vi "Prova_1.vi"(8 "error in (no error)":errorcluster, 11 "This VI":refnum<vi>) -> (0 "error out":errorcluster)   [LabVIEW 2016]
uses:
  USER32.DLL
  Program Files (x86)/VideoLAN/VLC/libvlc.dll
  System.Windows.Forms
panel:
  out "speed":dbl
  in  "PictureBox":refnum<k24>(container)
  in  "Script":string
  in  "Media Source":string="rtsp://admin:admin@192.168.1.108:554/cam/realmonitor?channel=1&subtype=1"
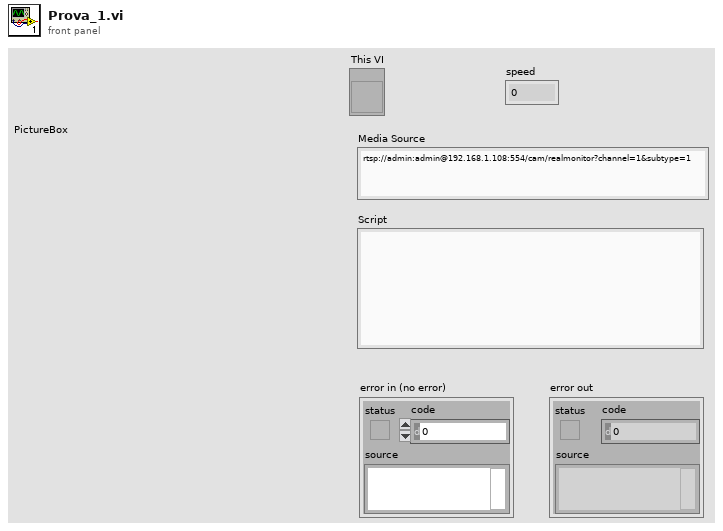
[diagram p1: front panel]
types:
  T1 = typedef "imagedata.ctl" = cluster{"image type":i32, "image depth":i32, "image":u8[], "mask":u8[], "colors":u32[], "Rectangle":cluster{"left":i16, "top":i16, "right":i16, "bottom":i16}}
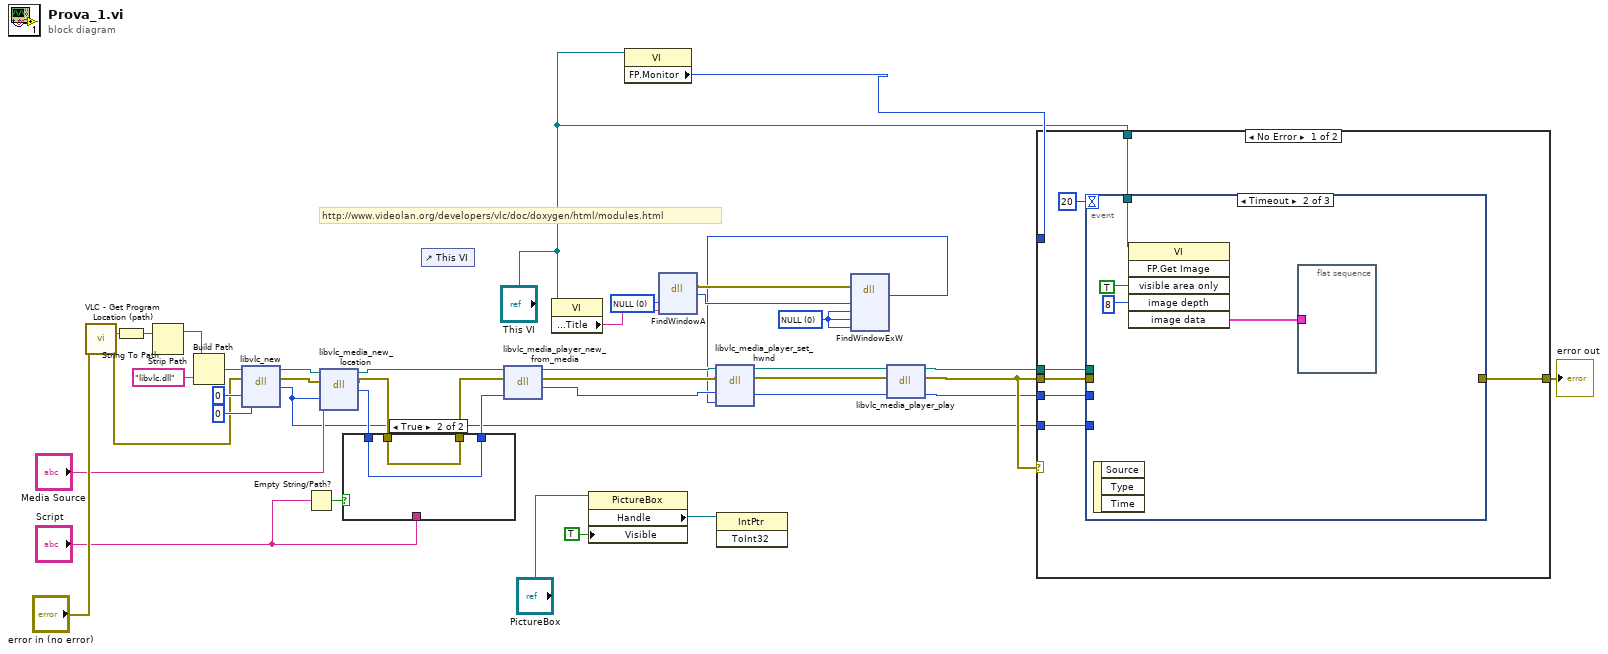
[diagram p0: block diagram]
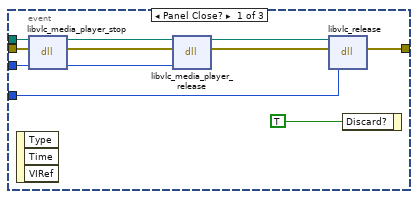
[diagram p2: hidden frame]
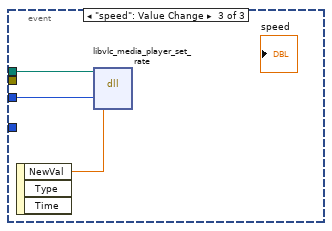
[diagram p3: hidden frame]
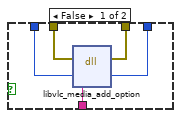
[diagram p5: hidden frame]
diagram:
  w4 = 0 items=["NULL"]
  w41 = 0 items=["NULL"]
  # "http://www.videolan.org/developers/vlc/doc/doxygen/html/modules.html"
  n1 = call "VLC - Get Program Location (path).vi"("error in (no error)"="error in (no error)") -> ("VLC path"=w37:string, "error out"=w31:errorcluster)  [unwired: 13 in]
  n2 = String To Path(string=w37) -> (path=w36:path)
  n3 = Strip Path(path=w36) -> (stripped path=w35:path)  [unwired: 1 out]
  n4 = Build Path(base path=w35, name or relative path="libvlc.dll") -> (appended path=w33:path)
  n5 = dll-call lib="C:/Program Files (x86)/VideoLAN/VLC/libvlc.dll" fn="libvlc_new"(path in=w33, error in=w31, "argc"=i16 0, "argv"=u8 0) -> (path out=w11:path, error out=w12:errorcluster, "return type"=w7:i32)  [unwired: 3 in]
  n6 = Empty String/Path?(string/path="Script") -> (empty?=w29:bool)
  n7 = dll-call lib="C:/Program Files (x86)/VideoLAN/VLC/libvlc.dll" fn="libvlc_media_new_location"(path in=w11, error in=w12, "p_instance"=w7, "path"="Media Source") -> (path out=w10:path, error out=w13:errorcluster, "return type"=w8:i32)  [unwired: 3 in]
  n8 = case shown="True" w29 {
    tunnel: w13 -> [w46 w48]
    tunnel: w8 -> [w45 w47]
    tunnel: [w44 w47] -> w17
    tunnel: [w43 w48] -> w18
    tunnel: "Script" -> [w42 _]
    frame False {
      n9 = dll-call lib="C:/Program Files (x86)/VideoLAN/VLC/libvlc.dll" fn="libvlc_media_add_option"(error in=w46, "p_md"=w45, "ppsz_options"=w42) -> (error out=w43:errorcluster, "p_md"=w44:i32)  [unwired: 4 in, 1 out]
    }
    frame True {
    }
  }
  n10 = control-ref of="This VI"() -> ()  [unwired: 1 out]
  n11 = dll-call lib="C:/Program Files (x86)/VideoLAN/VLC/libvlc.dll" fn="libvlc_media_player_new_from_media"(path in=w10, error in=w18, "p_md"=w17) -> (path out=w14:path, error out=w15:errorcluster, "return type"=w16:i32)  [unwired: 2 in]
  n12 = property class="VI"(reference="This VI") -> ("Front Panel.Title"=w40:string)  [unwired: 1 in, 2 out]
  n13 = property class="PictureBox"(reference="PictureBox", "Visible"=TRUE ("Enabled")) -> ("Handle"=w27:refnum<k24>)  [unwired: 1 in, 2 out]
  n14 = property class="VI"(reference="This VI") -> ("FP.Monitor"=w6:u16)  [unwired: 1 in, 2 out]
  n15 = dll-call lib="USER32.DLL" fn="FindWindowA" label="FindWindow"("lpszClassName"=w41, "lpszWindowName"=w40) -> (error out=w3:errorcluster, "hWnd"=w2:u32)  [unwired: 5 in, 1 out]
  n16 = invoke class="IntPtr" method="ToInt32"(reference=w27) -> ()  [unwired: 2 in, 3 out]
  n17 = dll-call lib="user32.dll" fn="FindWindowExW" label="FindWindowEx"(error in=w3, "hwndParent"=w2, "hwndChildAfter"=w4, "lpszClassName"=w4, "lpszWindowName"=w4) -> ("hWnd"=w1:u32)  [unwired: 6 in, 2 out]
  n18 = dll-call lib="C:/Program Files (x86)/VideoLAN/VLC/libvlc.dll" fn="libvlc_media_player_set_hwnd"(path in=w14, error in=w15, "p_mi"=w16, "drawable"=w1) -> (path out=w26:path, error out=w24:errorcluster, "p_mi"=w25:i32)  [unwired: 3 in]
  n19 = dll-call lib="C:/Program Files (x86)/VideoLAN/VLC/libvlc.dll" fn="libvlc_media_player_play"(path in=w26, error in=w24, "p_mi"=w25) -> (path out=w22:path, error out=w23:errorcluster, "p_mi"=w21:i32)  [unwired: 2 in]
  n20 = case shown="No Error" w23 {
    tunnel: w7 -> [w55 _]
    tunnel: w21 -> [w54 _]
    tunnel: w23 -> [w53 w74]
    tunnel: w22 -> [w52 _]
    tunnel: [w51 w74] -> w28
    tunnel: w6 -> [_ _]
    tunnel: "This VI" -> [w49 _]
    frame No Error {
      n21 = event shown="[1] Timeout" {
        selector: _ -> [_ _ _]
        dyn-events: _ -> [_ _ _]
        timeout: 20 -> [_ _ _]
        tunnel: w53 -> [w66 _ _]
        tunnel: w54 -> [w65 _ w71]
        tunnel: w55 -> [w61 _ _]
        tunnel: w52 -> [w59 _ w73]
        tunnel: [w56 _ _] -> w51
        tunnel: w49 -> [_ w70 _]
        event Panel Close? {
          n22 = event-data() -> ()  [unwired: 1 in, 3 out]
          n23 = dll-call lib="C:/Program Files (x86)/VideoLAN/VLC/libvlc.dll" fn="libvlc_media_player_stop"(path in=w59, error in=w66, "p_mi"=w65) -> (path out=w58:path, error out=w64:errorcluster, "p_mi"=w63:i32)  [unwired: 2 in]
          n24 = dll-call lib="C:/Program Files (x86)/VideoLAN/VLC/libvlc.dll" fn="libvlc_media_player_release"(path in=w58, error in=w64, "p_mi"=w63) -> (path out=w57:path, error out=w62:errorcluster)  [unwired: 3 in]
          n25 = dll-call lib="C:/Program Files (x86)/VideoLAN/VLC/libvlc.dll" fn="libvlc_release"(path in=w57, error in=w62, "p_instnace"=w61) -> (error out=w56:errorcluster)  [unwired: 3 in, 1 out]
          n26 = event-data("Discard?"=TRUE) -> ()  [unwired: 1 in, 1 out]
        }
        event Timeout {
          n27 = event-data() -> ()  [unwired: 1 in, 3 out]
          n28 = invoke class="VI" method="FP.Get Image"(reference=w70, "visible area only"=TRUE ("Visible Area Only"), "image depth"=8 ("Image Depth")) -> ("image data"=w69:T1)  [unwired: 3 in, 5 out]
          n29 = flat-sequence {
            tunnel: w69 -> [_]
            frame #0 {
            }
          }
        }
        event "speed": Value Change {
          n30 = event-data() -> ("NewVal"=w72:dbl)  [unwired: 1 in, 2 out]
          n31 = dll-call lib="C:/Program Files (x86)/VideoLAN/VLC/libvlc.dll" fn="libvlc_media_player_set_rate"(path in=w73, "p_mi"=w71, "rate"=w72) -> ()  [unwired: 5 in, 2 out]
        }
      }
    }
    frame Error {
    }
  }
  "error out" <- w28
